vi "DAQ_StopRecord.vi"(8 "error in (no error)":errorcluster, 9 "Label":string, 10 "Task":string, 11 "Message Enqueuer":refnum<class "Message Enqueuer.lvclass">) -> (0 "error out":errorcluster)   [LabVIEW 2025, in "DAQ_API.lvlib"]
uses:
  DAQ_API.lvlib
  <vilib>/ActorFramework/Message Enqueuer/Message Enqueuer.lvclass
  DAQ_Module/DAQ_Module/DAQ_Module Messages/StopRecord Msg/StopRecord Msg.lvclass/StopRecord Msg.ctl
  <vilib>/ActorFramework/Message Enqueuer/Message Enqueuer.lvclass/Message Enqueuer.ctl
  <vilib>/ActorFramework/Message Enqueuer/Enqueue.vi
  DAQ_Module/DAQ_Module/DAQ_Module Messages/StopRecord Msg/StopRecord Msg.lvclass
  C:/Program Files (x86)/National Instruments/LabVIEW 2025/vi.lib/ActorFramework/Message/Message.lvclass
  <vilib>/ActorFramework/Message Priority Queue/Priority Enqueue.vi
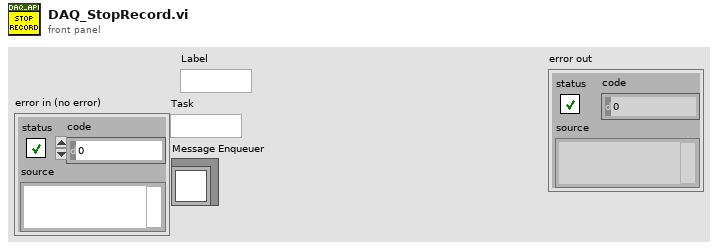
[diagram p1: front panel]
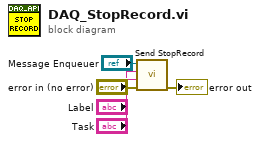
[diagram p0: block diagram]
diagram:
  n1 = call "Send StopRecord.vi"("error in (no error)"="error in (no error)", "Label"="Label", "Task"="Task", "Message Enqueuer"="Message Enqueuer") -> ("error out"=→"error out":errorcluster)  [unwired: 6 in, 1 out]
